vi "Construct_Log_File_Path.vi"(8 "error in (no error)":errorcluster, 10 "filename without extension":string, 11 "build":refnum<class "AB_DepSourceDist.lvclass">) -> (0 "error out":errorcluster, 3 "appended path":path)   [LabVIEW 2020, in "AB_DepSourceDist.lvclass"]
uses:
  <vilib>/AppBuilder/AB_Classes/DepSourceDist/AB_DepSourceDist.lvclass
  e:/builds/penguin/labview/branches/2020/dev/dist/vi.lib/AppBuilder/AB_Classes/Build/AB_Build.lvclass
  <vilib>/AppBuilder/AB_Classes/Deployment/AB_Deployment.lvlib
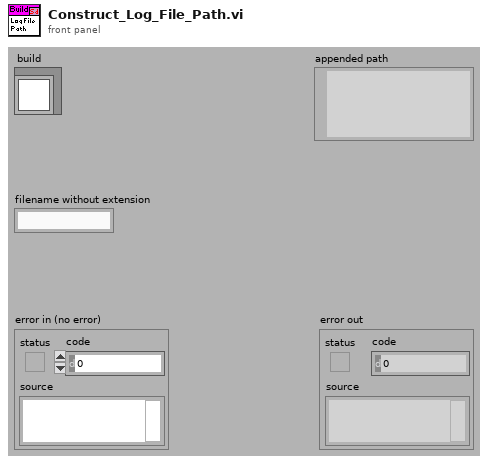
[diagram p1: front panel]
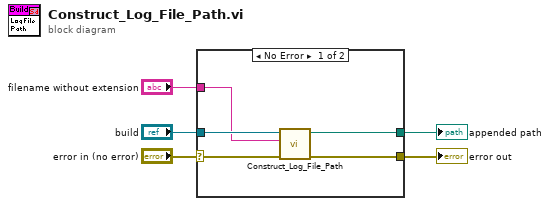
[diagram p0: block diagram]
diagram:
  n1 = case shown="No Error" "error in (no error)" {
    selector: "error in (no error)" -> [w8 w11]
    tunnel: "build" -> [w10 _]
    tunnel: [w9 _] -> w4
    tunnel: "filename without extension" -> [w6 _]
    tunnel: [w7 w11] -> w1
    frame No Error {
      n2 = call <vilib>:"Construct_Log_File_Path.vi"("error in (no error)"=w8, "filename without extension"=w6, "build"=w10) -> ("error out"=w7:errorcluster, "appended path"=w9:path)  [unwired: 7 in]
    }
    frame Error {
    }
  }
  "appended path" <- w4
  "error out" <- w1
